vi "UPDATE.vi"(6 "ANALOGICO/DIGITAL":bool, 8 "DAQ BOARD":tag, 9 "Adquisicion tiempo":i32, 10 "DIGITAL":T1={"Puertos Digital"=[], "Lineas Digital"=[], "Frecuencia Muestreo"=1000, "Puerto/Linea"=FALSE}, 11 "ANALOGICO":T2={"ANALOGICO CANALES"=[], "Numero de muestras"=1000, "Frecuencia de muestreo"=1000}) -> (0 "error out":errorcluster)   [LabVIEW 2020, in "Settings.lvlib"]
uses:
  Settings.lvlib
  Acquisition/cluster analogico.ctl
  Acquisition/cluster digital.ctl
  <vilib>/drjdpowell/SQLite Library/SQL Connection/Open (path).vi
  <vilib>/drjdpowell/SQLite Library/SQL Connection/Open (string).vi
  <vilib>/AdvancedString/Path To Command Line String.vi
  <vilib>/drjdpowell/SQLite Library/SQL Connection/Execute SQL (No results).vi
  <vilib>/drjdpowell/SQLite Library/SQL Connection/Connection.lvclass
  <vilib>/drjdpowell/SQLite Library/SQLite.lvlib
  Acquisition/CONTROLS.lvlib
panel:
  in  "error in (no error)":errorcluster
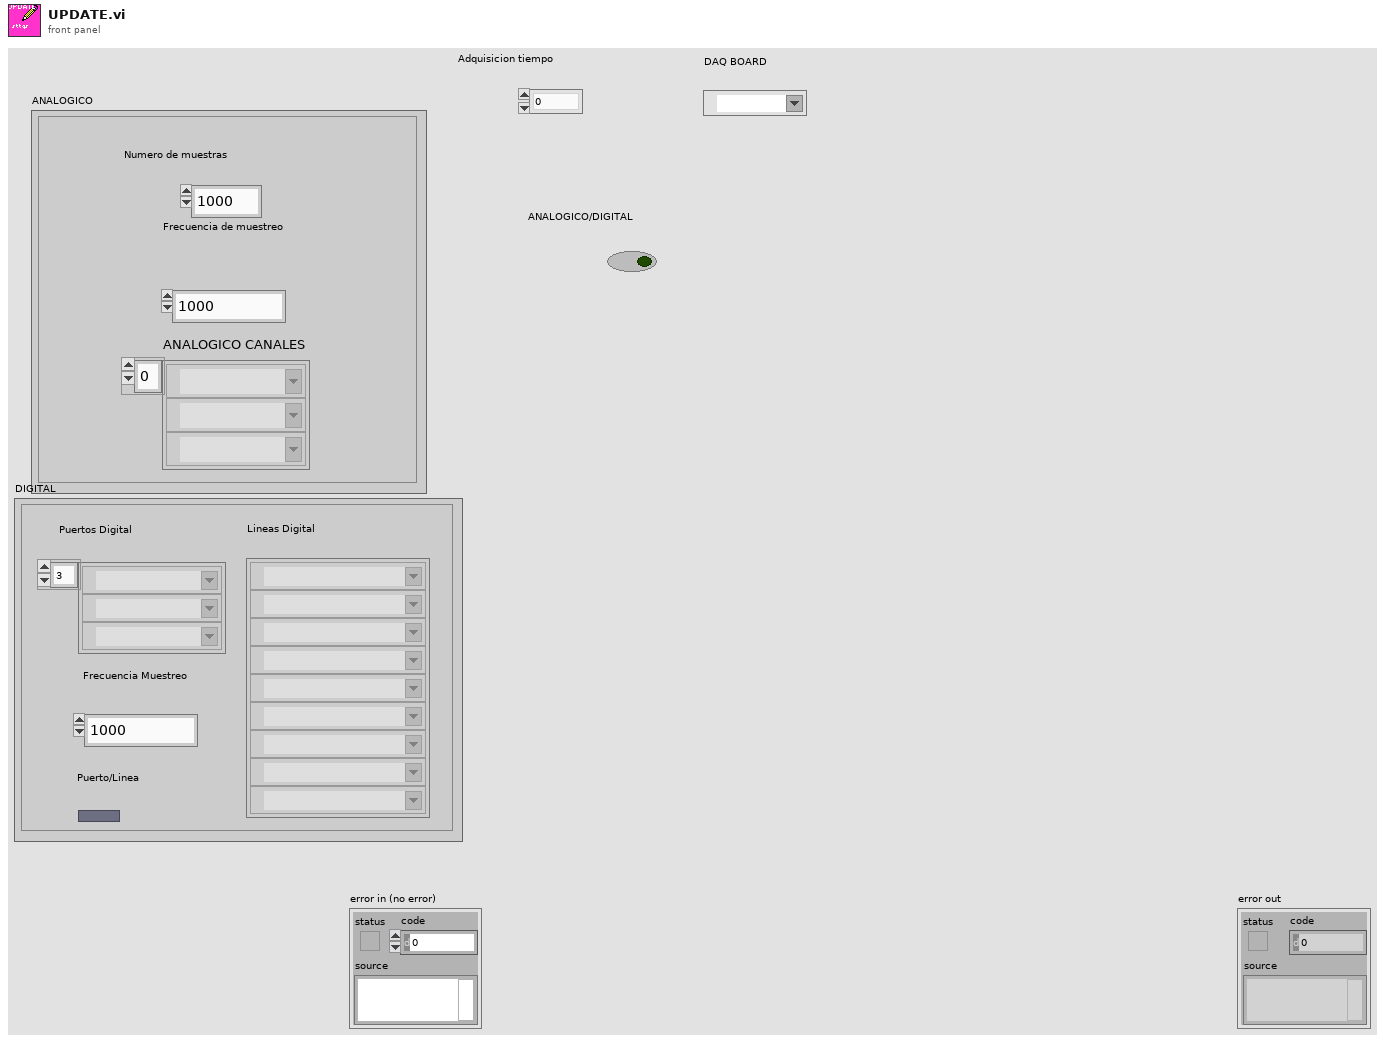
[diagram p1: front panel]
types:
  T1 = typedef "Acquisition.lvlib/CONTROLS.lvlib/cluster digital.ctl" = cluster{"Puertos Digital":tag[], "Lineas Digital":tag[], "Frecuencia Muestreo":u32, "Puerto/Linea":bool}
  T2 = typedef "Acquisition.lvlib/CONTROLS.lvlib/cluster analogico.ctl" = cluster{"ANALOGICO CANALES":tag[], "Numero de muestras":u32, "Frecuencia de muestreo":u32}
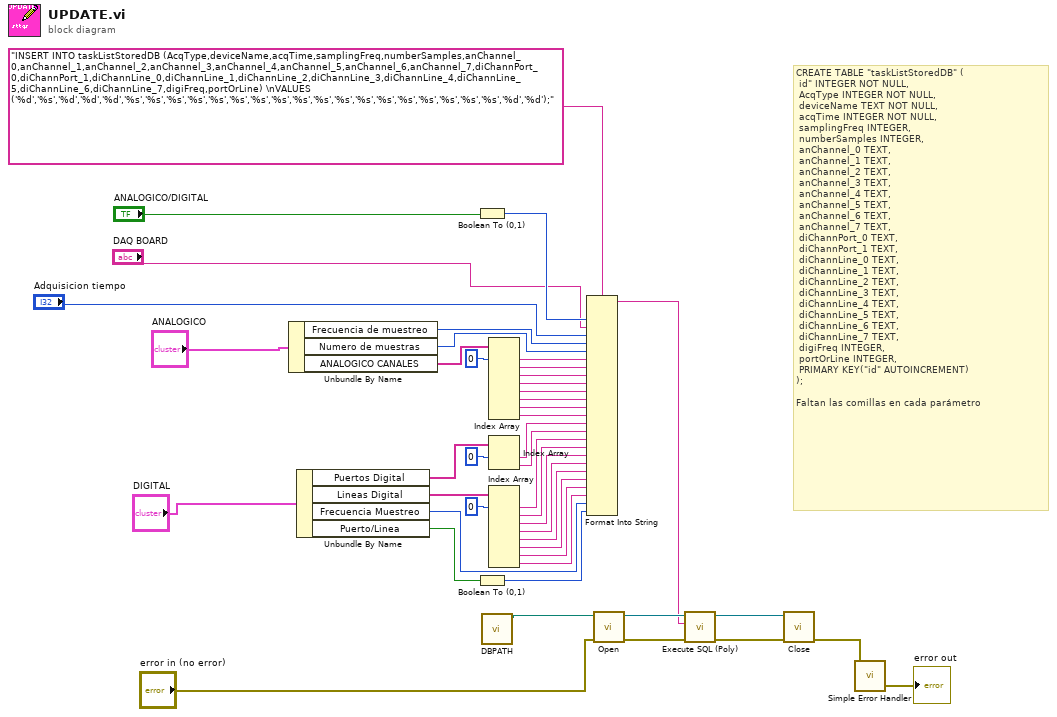
[diagram p0: block diagram]
diagram:
  # "CREATE TABLE \"taskListStoredDB\" (\n\tid\"\tINTEGER NOT NULL,\n\tAcqType\tINTEGER NOT NULL,\n\tdeviceName\tTEXT NOT NULL,\n\tacqTime\tINTEGER NOT NULL,\n\tsamplingFreq\tINTEGER,\n\tnumberSamples\tINTEGER,\n\tanChannel_0\tTEXT,\n\tanChannel_1\tTEXT,\n\tanChannel_2\tTEXT,\n\tanChannel_3\tTEXT,\n\tanChannel_4 TEXT,\n\tanChannel_5\tTEXT,\n\tanChannel_6\tTEXT,\n\tanChannel_7\tTEXT,\n\tdiChannPort_0\tTEXT,\n\tdiChannPort_1\tTEXT,\n\tdiChannLine_0\tTEXT,\n\tdiChannLine_1\tTEXT,\n\tdiChannLine_2\tTEXT,\n\tdiChannLine_3\tTEXT,\n\tdiChannLine_4\tTEXT,\n\tdiChannLine_5\tTEXT,\n\tdiChannLine_6\tTEXT,\n\tdiChannLine_7\tTEXT,\n\tdigiFreq\tINTEGER,\n\tportOrLine INTEGER,\n\tPRIMARY KEY(\"id\" AUTOINCREMENT)\n);\n\nFaltan las comillas en cada parámetro"
  n1 = Unbundle By Name("ANALOGICO") -> ("Frecuencia de muestreo"=w43:u32, "Numero de muestras"=w42:u32, "ANALOGICO CANALES"=w40:tag[])
  n2 = Unbundle By Name("DIGITAL") -> ("Puertos Digital"=w30:tag[], "Lineas Digital"=w26:tag[], "Frecuencia Muestreo"=w17:u32, "Puerto/Linea"=w16:bool)
  n3 = Boolean To (0,1)(Boolean="ANALOGICO/DIGITAL") -> (0, 1=w44:i16)
  n4 = Boolean To (0,1)(Boolean=w16) -> (0, 1=w15:i16)
  n5 = call "DBPATH.vi"() -> ("appended path"=w5:path)  [unwired: 11 in]
  n6 = Index Array(array=w40, index #1=0 ("index")) -> (element #1=w39:tag, element #2=w38:tag, element #3=w37:tag, element #4=w36:tag, element #5=w35:tag, element #6=w34:tag, element #7=w33:tag, element #8=w32:tag)  [unwired: 7 in]
  n7 = Index Array(array=w30, index #1=0 ("index")) -> (element #1=w29:tag, element #2=w28:tag)  [unwired: 1 in]
  n8 = Index Array(array=w26, index #1=0 ("index")) -> (element #1=w25:tag, element #2=w24:tag, element #3=w23:tag, element #4=w22:tag, element #5=w21:tag, element #6=w20:tag, element #7=w19:tag, element #8=w18:tag)  [unwired: 7 in]
  n9 = Format Into String(format string="INSERT INTO taskListStoredDB (AcqType,deviceName,acqTime,samplingFreq,numberSamples,anChannel_0,anChannel_1,anChannel_2,anChannel_3,anChannel_4,anChannel_5,anChannel_6,anChannel_7,diChannPort_0,diChannPort_1,diChannLine_0,diChannLine_1,diChannLine_2,diChannLine_3,diChannLine_4,diChannLine_5,diChannLine_6,diChannLine_7,digiFreq,portOrLine) \nVALUES ('%d','%s','%d','%d','%d','%s','%s','%s','%s','%s','%s','%s','%s','%s','%s','%s','%s','%s','%s','%s','%s','%s','%s','%d','%d');", w44, "DAQ BOARD", "Adquisicion tiempo", w43, w42, w39, w38, w37, w36, w35, w34, w33, w32, w29, w28, w25, w24, w23, w22, w21, w20, w19, w18, w17, w15) -> (resulting string=w9:string)  [unwired: 2 in, 1 out]
  n10 = call-poly <vilib>:"Open.vi"("error in (no error)"="error in (no error)", "db file"=w5) -> ("error out"=w14:errorcluster, "SQLite Connection"=w11:refnum<class "Connection.lvclass">)  [unwired: 8 in]
  n11 = call-poly <vilib>:"Execute SQL (Poly).vi"("error in (no error)"=w14, "SQL"=w9, "SQLite Connection in"=w11) -> ("error out"=w12:errorcluster, "SQLite Connection"=w13:refnum<class "Connection.lvclass">)  [unwired: 7 in]
  n12 = call-dynamic "Close.vi"("error in (no error)"=w12, "SQLite Connection in"=w13) -> ("error out"=w8:errorcluster)  [unwired: 9 in]
  n13 = call <vilib>:"Simple Error Handler.vi"("error in (no error)"=w8) -> ("error out"=→"error out":errorcluster)  [unwired: 4 in, 4 out]
